vi "From JSON String.vi"(0 "Display State In":T1, 7 "JSON String":string, 9 "Container State":T2, 11 "error in (no error)":errorcluster) -> (4 "Display State Out":T1, 15 "error out":errorcluster)   [LabVIEW 2017, in "Advanced Variant Tools.lvlib" / "Variant Tree.xctl"]
uses:
  Variant Tree.xctl
  <vilib>/_xctls/Container State.ctl
  State.ctl
  Variant JSON API/Source/Variant JSON API.lvlib
  <vilib>/_xctls/XControlSupport.lvlib
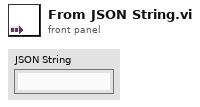
[diagram p1: front panel]
types:
  T1 = typedef "Advanced Variant Tools.lvlib/Variant Tree.xctl/State.ctl" = cluster{"Numeric":dbl}
  T2 = typedef "XControlSupport.lvlib/Container State.ctl" = cluster{"Indicator?":bool, "Run Mode?":bool, " Refnum":refnum<vi>}
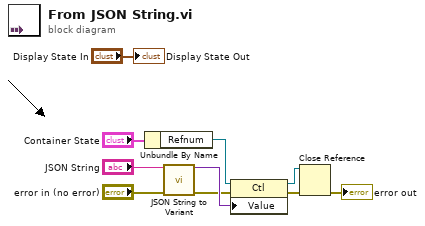
[diagram p0: block diagram]
diagram:
  n1 = Unbundle By Name("Container State") -> ("Refnum"=w8:refnum<vi>)
  n2 = call "JSON String to Variant.vi"("JSON String"="JSON String", "error in (no error)"="error in (no error)") -> ("Variant out"=w7:variant, "error out"=w4:errorcluster)  [unwired: 12 in]
  n3 = property class="Ctl"(reference=w8, error in=w4, "Value"=w7) -> (reference out=w1:refnum<vi>, error out=w3:errorcluster)
  n4 = Close Reference(reference=w1, error in (no error)=w3) -> (error out=→"error out":errorcluster)
  "Display State Out" <- "Display State In"
